vi "Keithley6485 Read.vi"(7 "Enable Zero Correction":bool=TRUE, 8 "error in":errorcluster, 10 "Sample per measurement":u32=1 max=2500, 11 "VISA in":refnum<visa-resource-name>="COM3") -> (0 "error out":errorcluster, 1 "Zero Offset":string, 2 "Current (A)":dbl, 3 "VISA out":refnum<visa-resource-name>)   [LabVIEW 2018]
uses:
  <vilib>/Analysis/baseanly.llb/Mean (DBL).vi
  <vilib>/Analysis/NI_AALBase.lvlib
panel:
  in  "Zero Correction Procedure":string=":TRIG:COUN 1;:SYST:ZCH 1;:CURR:RANG 2E-9;:INIT;:SYST:ZCOR:ACQ;:SYST:ZCH 0;:SYST:ZCOR 1;:CURR:RANG:AUTO 1;FETC?"
  in  "Error procedure":string
  out "read buffer":string
  in  "Bytes to Read":i32=40000
  # "Error out reports Serial I/O errors.\n\nKeithley Error reports error messages returned by the Keithley 6485 picoAmmeter.  Currently, only overvoltage and invalid data errors are supported by this VI."
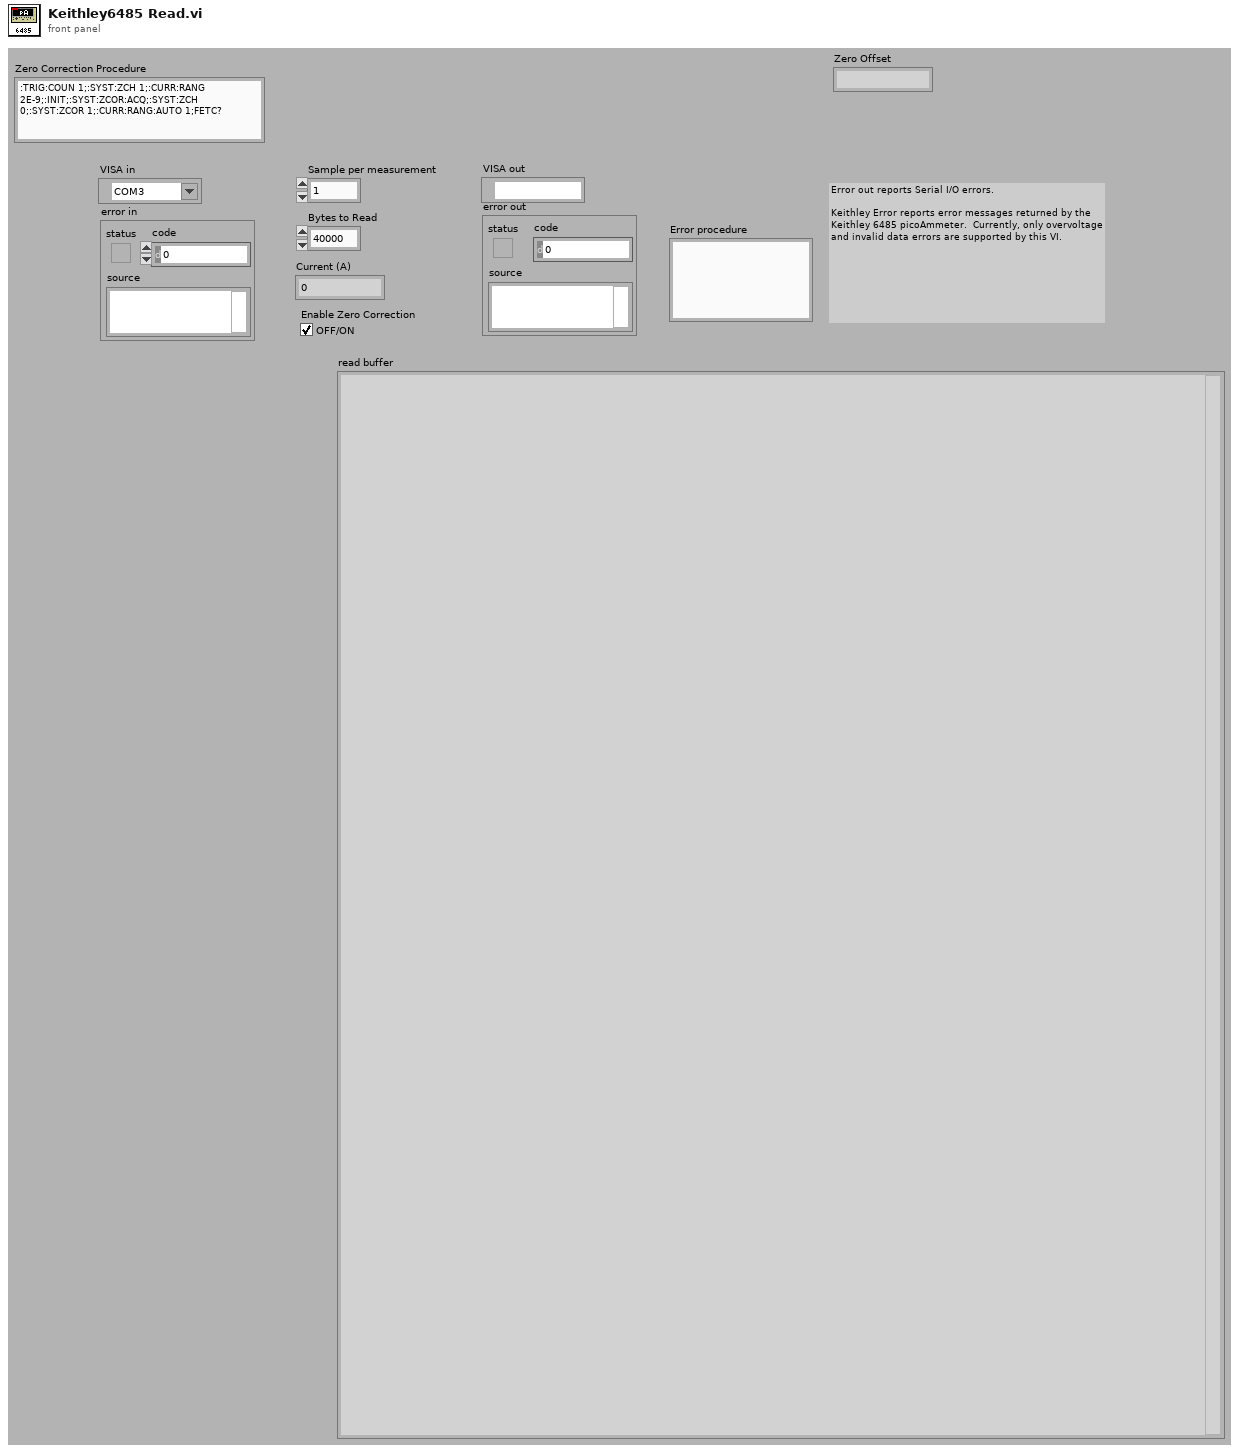
[diagram p1: front panel]
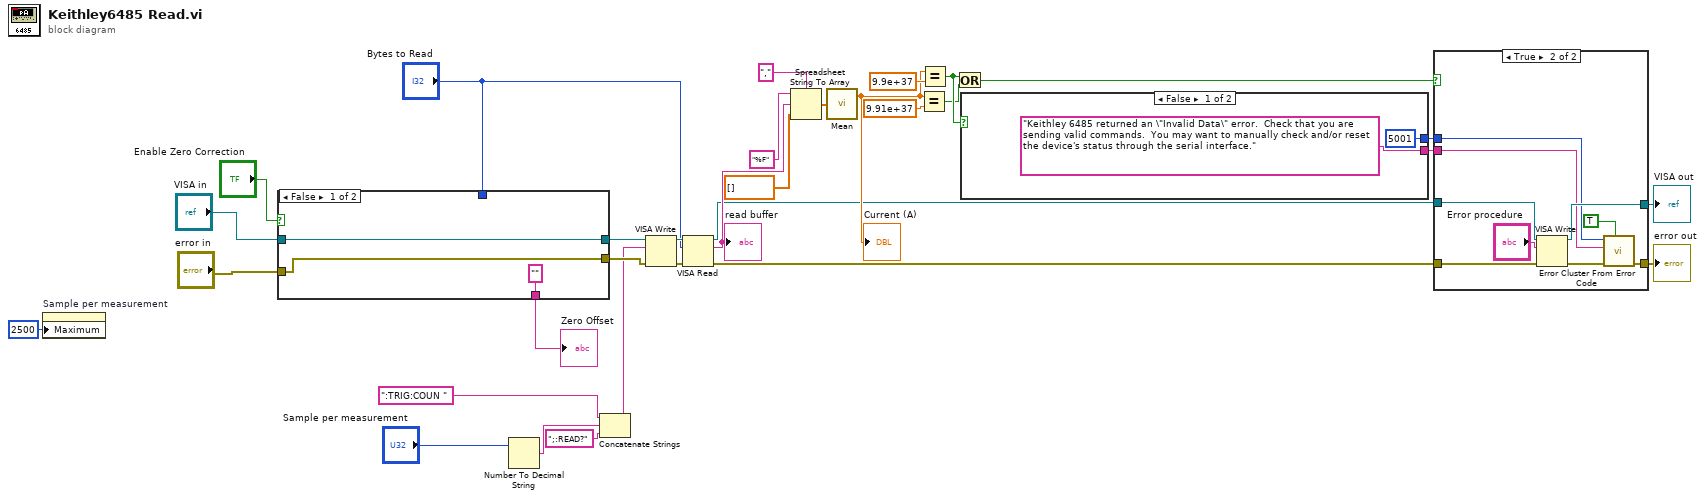
[diagram p0: block diagram]
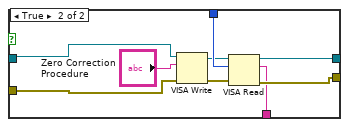
[diagram p2: hidden frame]
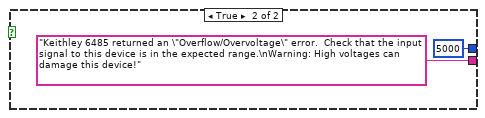
[diagram p3: hidden frame]
diagram:
  n1 = property on="Sample per measurement" class="DigNum (strict)"("Maximum"=u32 2500 ("Data Entry Limits:Maximum")) -> ()  [unwired: 2 in, 2 out]
  n2 = case shown="False" "Enable Zero Correction" {
    tunnel: "VISA in" -> [w35 w43]
    tunnel: "error in" -> [w34 w42]
    tunnel: "Bytes to Read" -> [_ w41]
    tunnel: [w34 w38] -> w3
    tunnel: [w35 w37] -> w4
    tunnel: ["" ("read buffer") w36] -> w2
    frame False {
    }
    frame True {
      n3 = VISA Write(VISA resource name=w43, write buffer="Zero Correction Procedure", error in (no error)=w42) -> (VISA resource name out=w40:refnum<visa-resource-name>, error out=w39:errorcluster)  [unwired: 1 out]
      n4 = VISA Read(VISA resource name=w40, byte count=w41, error in (no error)=w39) -> (VISA resource name out=w37:refnum<visa-resource-name>, read buffer=w36:string, error out=w38:errorcluster)  [unwired: 1 out]
    }
  }
  "Zero Offset" <- w2
  n5 = Number To Decimal String(number="Sample per measurement") -> (decimal integer string=w29:string)  [unwired: 1 in]
  n6 = Concatenate Strings(":TRIG:COUN ", w29, ";:READ?") -> (w1:string)
  n7 = VISA Write(VISA resource name=w4, write buffer=w1, error in (no error)=w3) -> (VISA resource name out=w31:refnum<visa-resource-name>, error out=w32:errorcluster)  [unwired: 1 out]
  n8 = VISA Read(VISA resource name=w31, byte count="Bytes to Read", error in (no error)=w32) -> (VISA resource name out=w17:refnum<visa-resource-name>, read buffer=w26:string, error out=w16:errorcluster)  [unwired: 1 out]
  "read buffer" <- w26
  n9 = Spreadsheet String To Array(delimiter (Tab)=",", format string="%F", spreadsheet string=w26, array type (2D Dbl)=dbl[] [] ("Array")) -> (array=w23:dbl[])
  n10 = call-poly <vilib>:"Mean.vi"("X"=w23) -> ("mean"=w18:dbl)  [unwired: 1 out]
  "Current (A)" <- w18
  n11 = Equal?(x=w18, y=9.91e+37) -> (x = y?=w12:bool)
  n12 = Equal?(x=w18, y=9.9e+37) -> (x = y?=w13:bool)
  n13 = Or(x=w13, y=w12) -> (x .or. y?=w14:bool)
  n14 = case shown="False" w13 {
    tunnel: ["Keithley 6485 returned an \"Invalid Data\" error.  Check that you are sending valid commands.  You may want to manually check and/or reset the device's status through the serial interface." "Keithley 6485 returned an \"Overflow/Overvoltage\" error.  Check that the input signal to this device is in the expected range.\nWarning: High voltages can damage this device!"] -> w9
    tunnel: [5001 ("error code (0)") 5000 ("error code (0)")] -> w8
    frame False {
    }
    frame True {
    }
  }
  n15 = case shown="True" w14 {
    tunnel: w17 -> [w50 w59]
    tunnel: w16 -> [w49 w58]
    tunnel: [w50 w57] -> w15
    tunnel: [w49 w54] -> w10
    tunnel: w9 -> [_ w53]
    tunnel: w8 -> [_ w51]
    frame False {
    }
    frame True {
      n16 = VISA Write(VISA resource name=w59, write buffer="Error procedure", error in (no error)=w58) -> (VISA resource name out=w57:refnum<visa-resource-name>, error out=w55:errorcluster)  [unwired: 1 out]
      n17 = call <vilib>:"Error Cluster From Error Code.vi"("show call chain? (False)"=TRUE, "error in (no error)"=w55, "error message (\"\")"=w53, "error code (0)"=w51) -> ("error out"=w54:errorcluster)  [unwired: 5 in]
    }
  }
  "VISA out" <- w15
  "error out" <- w10
